vi "TheilSenRegressor.vi"(8 "error in":errorcluster) -> (0 "error out":errorcluster, 3 "out":refnum<class "TheilSenRegressor.lvclass">)   [LabVIEW 2020]
doc: "Theil-Sen Estimator: robust multivariate regression model.\n\n The algorithm calculates least square solutions on subsets with size\n n_subsamples of the samples in X. Any value of n_subsamples between the\n number of features and samples leads to an estimator with a compromise\n between robustness and efficiency. Since the number of least square\n solutions is \"n_samples choose n_subsamples\", it can be extremely large\n and can therefore be limited with max_subpopulation. If this limit is\n reached, the subsets are chosen randomly. In a final step, the spatial\n median (or L1 median) is calculated of all least square solutions.\n\n Read more in the :ref:`User Guide <theil_sen_regression>`.\n\n Parameters\n ----------\n fit_intercept : bool, default=True\n Whether to calculate the intercept for this model. If set\n to false, no intercept will be used in calculations.\n\n copy_X : bool, default=True\n If True, X will be copied; else, it may be overwritten.\n\n max_subpopulation : int, default=1e4\n Instead of computing with a set of cardinality 'n choose k', where n is\n the number of samples and k is the number of subsamples (at least\n number of features), consider only a stochastic subpopulation of a\n given maximal size if 'n choose k' is larger than max_subpopulation.\n For other than small problem sizes this parameter will determine\n memory usage and runtime if n_subsamples is not changed.\n\n n_subsamples : int, default=None\n Number of samples to calculate the parameters. This is at least the\n number of features (plus 1 if fit_intercept=True) and the number of\n samples as a maximum. A lower number leads to a higher breakdown\n point and a low efficiency while a high number leads to a low\n breakdown point and a high efficiency. If None, take the\n minimum number of subsamples leading to maximal robustness.\n If n_subsamples is set to n_samples, Theil-Sen is identical to least\n squares.\n\n max_iter : int, default=300\n Maximum number of iterations for the calculation of spatial median.\n\n tol : float, default=1.e-3\n Tolerance when calculating spatial median.\n\n random_state : int, RandomState instance or None, default=None\n A random number generator instance to define the state of the random\n permutations generator. Pass an int for reproducible output across\n multiple function calls.\n See :term:`Glossary <random_state>`\n\n n_jobs : int, default=None\n Number of CPUs to use during the cross validation.\n ``None`` means 1 unless in a :obj:`joblib.parallel_backend` context.\n ``-1`` means using all processors. See :term:`Glossary <n_jobs>`\n for more details.\n\n verbose : bool, default=False\n Verbose mode when fitting the model.\n\n Attributes\n ----------\n coef_ : ndarray of shape (n_features,)\n Coefficients of the regression model (median of distribution).\n\n intercept_ : float\n Estimated intercept of regression model.\n\n breakdown_ : float\n Approximated breakdown point.\n\n n_iter_ : int\n Number of iterations needed for the spatial median.\n\n n_subpopulation_ : int\n Number of combinations taken into account from 'n choose k', where n is\n the number of samples and k is the number of subsamples.\n\n \nAvailable methods:\nGet Attributes\nGet Params\nSet Params"
uses:
  TheilSenRegressor.lvclass
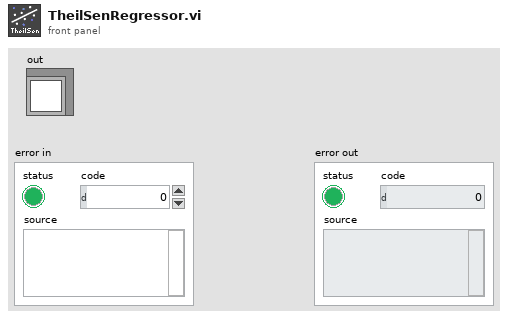
[diagram p1: front panel]
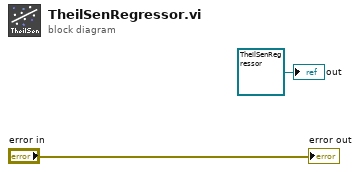
[diagram p0: block diagram]
diagram:
  "out" <- refnum<class "TheilSenRegressor.lvclass"> refnum ("model")
  "error out" <- "error in"
